vi "_iWorx - Drop Counter.vi"() -> ()   [LabVIEW 2012]
uses:
  <vilib>/DAQmx/create/channels.llb/DAQmx Create Channel (AI-Voltage-Basic).vi
  <vilib>/DAQmx/configure/timing.llb/DAQmx Timing (Sample Clock).vi
  <vilib>/DAQmx/read.llb/DAQmx Read (Analog 1D Wfm NChan NSamp).vi
panel:
  in  "Stop":bool
  in  "Log Info Button":bool
  out "Drop Count":u32
  in  "Reset count (f)":bool
  in  "Threshold":dbl format="%.2f"
  in  "Set Up":bool
  in  "Channel":u16(ring) items=["Channel 1", "Channel 2"]
  in  "Pause Button":bool
  in  "Snapshot":bool
  out "Waveform Chart":waveform(dbl)(graph)
  in  "Clear Chart":bool
  in  "Open Log":bool
  out "Raw Signal":dbl(knob) scale=-5.0..5.0
  # "iWorx - Drop Counter - Data Logger"
  # "Sensor Input"
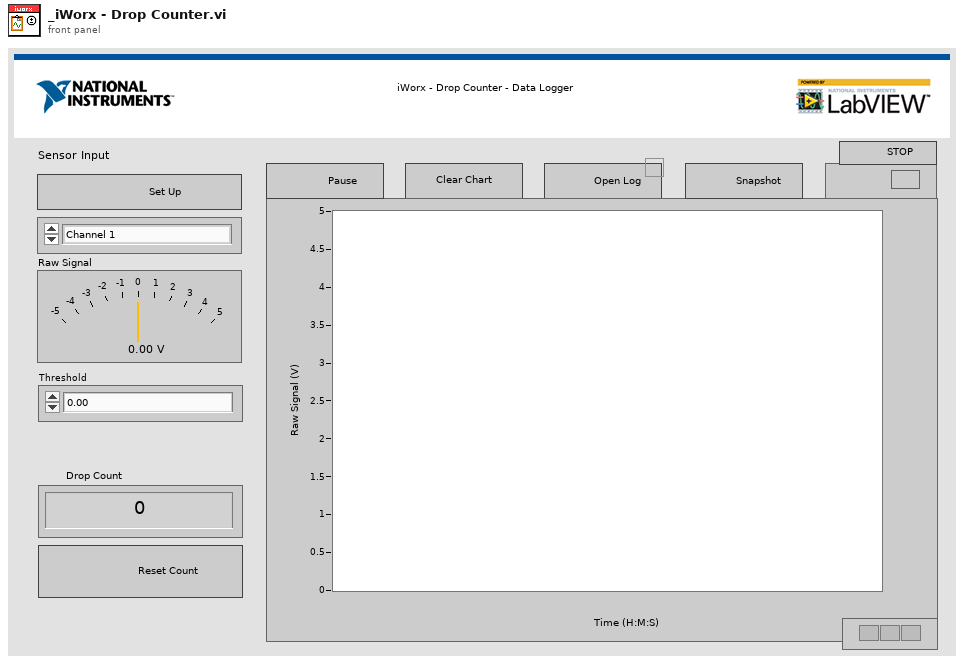
[diagram p1: front panel]
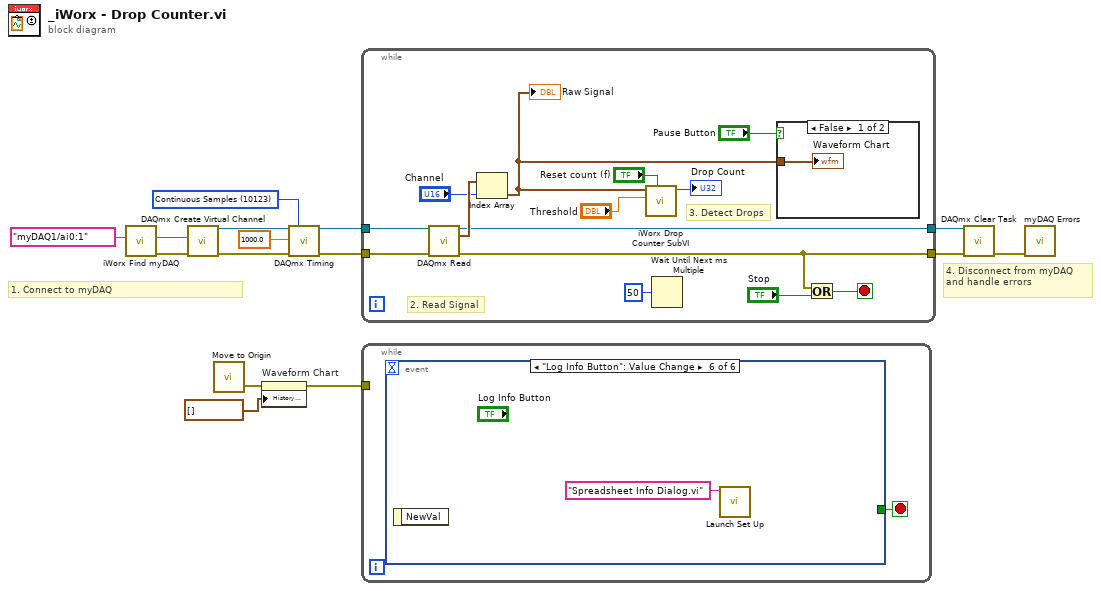
[diagram p0: block diagram]
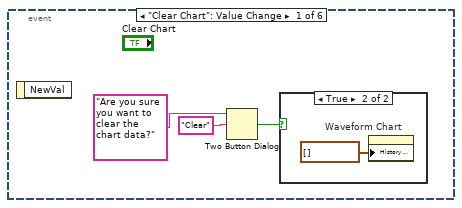
[diagram p2: hidden frame]
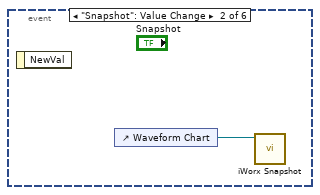
[diagram p4: hidden frame]
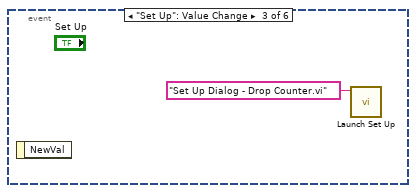
[diagram p5: hidden frame]
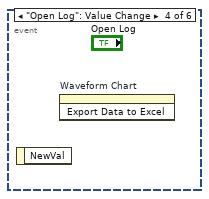
[diagram p6: hidden frame]
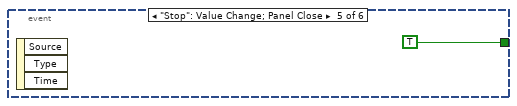
[diagram p7: hidden frame]
diagram:
  w7 = 10123 items=["Finite Samples"=10178, "Continuous Samples"=10123, "Hardware Timed Single Point"=12522] ("sample mode")
  # "4. Disconnect from myDAQ and handle errors"
  # "1. Connect to myDAQ"
  n1 = call "iWorx Find myDAQ.vi"("Preferred myDAQ (myDAQ1)"=tag "myDAQ1/ai0:1" ("physical channels")) -> ("Error Out"=w4:errorcluster, "DAQmx Physical Channel"=w3:tag)  [unwired: 6 in, 3 out]
  n2 = call-poly <vilib>:"DAQmx Create Virtual Channel.vi"("physical channels"=w3, "error in"=w4) -> ("task out"=w11:refnum<k21>, "error out"=w9:errorcluster)  [unwired: 12 in]
  n3 = call "Move to Origin.vi"() -> ("Error Out"=w5:errorcluster)  [unwired: 3 in]
  n4 = property on="Waveform Chart" class="WFChart (strict)"(error in=w5, "History Data"=waveform(dbl)[] []) -> (error out=w13:errorcluster)  [unwired: 1 in, 1 out]
  n5 = call-poly <vilib>:"DAQmx Timing.vi"("task/channels in"=w11, "sample mode"=w7, "rate"=1000.0, "error in"=w9) -> ("task out"=w10:refnum<k21>, "error out"=w8:errorcluster)  [unwired: 10 in]
  n6 = while {
    tunnel: w10 -> [w29]
    tunnel: [w22] -> w15
    tunnel: w8 -> [w28]
    tunnel: [w26] -> w14
    stop <- w27 stop-if-true
    # "3. Detect Drops"
    # "2. Read Signal"
    n7 = call-poly <vilib>:"DAQmx Read.vi"("task/channels in"=w29, "error in"=w28) -> ("task out"=w22:refnum<k21>, "data"=w24:waveform(dbl)[], "error out"=w26:errorcluster)  [unwired: 11 in]
    n8 = Index Array(array=w24, index="Channel") -> (element=w21:waveform(dbl))
    "Raw Signal" <- w21
    n9 = call "iWorx Drop Counter SubVI.vi"("Reset count (f)"="Reset count (f)", "Threshold (0V)"="Threshold", "waveform in"=w21) -> ("Drop Count"=→"Drop Count":u32)  [unwired: 5 in, 3 out]
    n10 = Wait Until Next ms Multiple(millisecond multiple=u32 50) -> ()  [unwired: 1 out]
    n11 = case shown="False" "Pause Button" {
      tunnel: w21 -> [w30 _]
      frame False {
        "Waveform Chart" <- w30
      }
      frame True {
      }
    }
    n12 = Or(x=w26, y="Stop") -> (x .or. y?=w27:bool)
  }
  n13 = while {
    tunnel: w13 -> [_]
    stop <- w31 stop-if-true
    n14 = event shown="[5] \"Log Info Button\": Value Change" {
      selector: _ -> [_ _ _ _ _ _]
      dyn-events: _ -> [_ _ _ _ _ _]
      timeout: _ -> [_ _ _ _ _ _]
      tunnel: [_ _ _ _ TRUE _] -> w31
      event "Clear Chart": Value Change {
        n15 = event-data() -> ()  [unwired: 1 in, 1 out]
        n16 = Two Button Dialog(message="Are you sure you want to clear the chart data?", 2:"Clear" ("T button name (\"OK\")")) -> (T button?=w33:bool)  [unwired: 1 in]
        n17 = case shown="True" w33 {
          frame False {
          }
          frame True {
            n18 = property on="Waveform Chart" class="WFChart (strict)"("History Data"=waveform(dbl)[] []) -> ()  [unwired: 2 in, 2 out]
          }
        }
      }
      event "Snapshot": Value Change {
        n19 = event-data() -> ()  [unwired: 1 in, 1 out]
        n20 = control-ref of="Waveform Chart"() -> (w36:refnum<vi>)
        n21 = call "iWorx Snapshot.vi"("WaveformChart in"=w36) -> ()  [unwired: 10 in, 1 out]
      }
      event "Set Up": Value Change {
        n22 = event-data() -> ()  [unwired: 1 in, 1 out]
        n23 = call "Launch Set Up.vi"("name or relative path"="Set Up Dialog - Drop Counter.vi") -> ()  [unwired: 9 in, 2 out]
      }
      event "Open Log": Value Change {
        n24 = event-data() -> ()  [unwired: 1 in, 1 out]
        n25 = invoke on="Waveform Chart" class="WFChart (strict)" method="Export Data to Excel"() -> ()  [unwired: 3 in, 3 out]
      }
      event "Stop": Value Change; Panel Close {
        n26 = event-data() -> ()  [unwired: 1 in, 3 out]
      }
      event "Log Info Button": Value Change {
        n27 = event-data() -> ()  [unwired: 1 in, 1 out]
        n28 = call "Launch Set Up.vi"("name or relative path"="Spreadsheet Info Dialog.vi") -> ()  [unwired: 9 in, 2 out]
      }
    }
  }
  n29 = call <vilib>:"DAQmx Clear Task.vi"("task in"=w15, "error in"=w14) -> ("error out"=w1:errorcluster)  [unwired: 13 in]
  n30 = call "myDAQ Errors.vi"("error in (no error)"=w1) -> ()  [unwired: 10 in, 1 out]
